vi "test.vi"() -> ()   [LabVIEW 2014]
panel:
  in  "stop":bool
  out "standard output":string
  out "standard error":string
  out "return code":i32
  out "error out":errorcluster
  in  "command line":string
  in  "standard input":string
  in  "working directory":path=path ""
  in  "error in (no error)":errorcluster
  in  "wait until completion? (T)":bool=TRUE
  in  "run minimized? (F)":bool
  in  "expected output size  (4096)":u32=4096
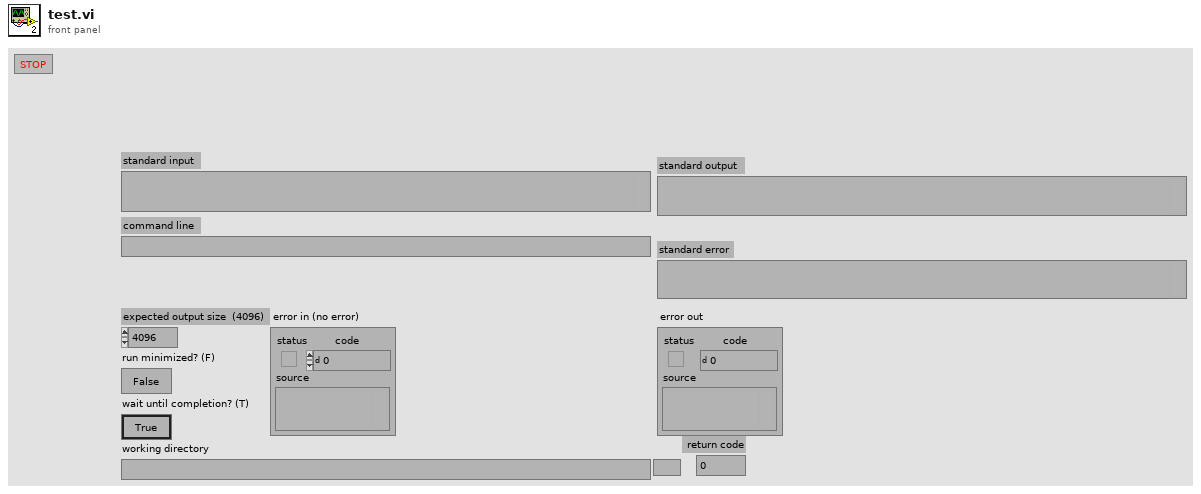
[diagram p1: front panel]
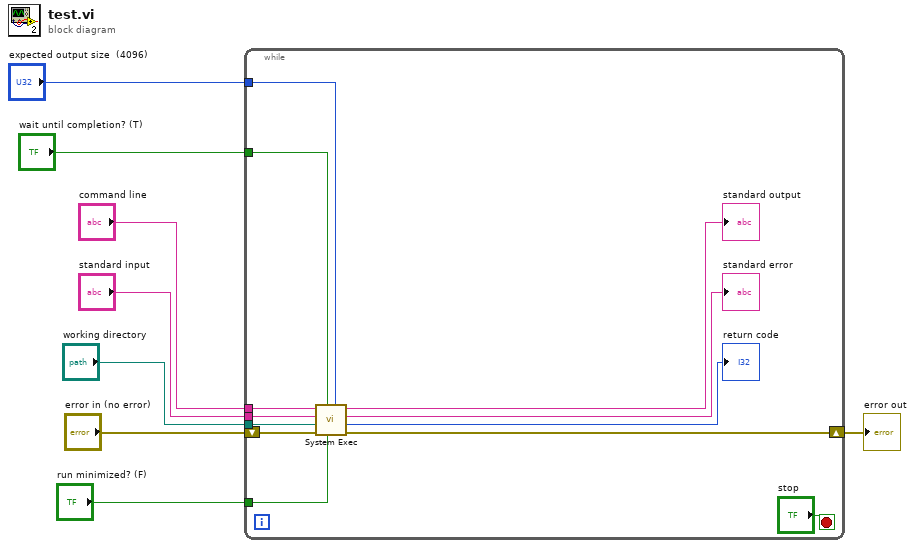
[diagram p0: block diagram]
diagram:
  n1 = while {
    tunnel: "expected output size  (4096)" -> [w20]
    tunnel: "run minimized? (F)" -> [w19]
    tunnel: "wait until completion? (T)" -> [w18]
    tunnel: "working directory" -> [w16]
    tunnel: "standard input" -> [w15]
    tunnel: "command line" -> [w14]
    shift-right: [w9] -> w1
    shift-left: "error in (no error)" -> [w17]
    stop <- "stop" stop-if-true
    n2 = call <vilib>:"System Exec.vi"("expected output size  (4096)"=w20, "run minimized? (F)"=w19, "wait until completion? (T)"=w18, "error in (no error)"=w17, "working directory"=w16, "standard input"=w15, "command line"=w14) -> ("error out"=w9:errorcluster, "return code"=→"return code":i32, "standard error"=→"standard error":string, "standard output"=→"standard output":string)  [unwired: 1 in]
  }
  "error out" <- w1
